vi "QAM Bit Grouping.vi"(1 "BitStream In":i32[](array[numeric]), 2 "QAM Complexity":T1(ring)) -> (0 "Symbol Out":i32[](array[numeric]))   [LabVIEW 2018]
doc: "Converts a binary stream into integer weights for QAM Modulation\nSupports: BPSK, QPSK, 16-QAM, 64-QAM, 256-QAM"
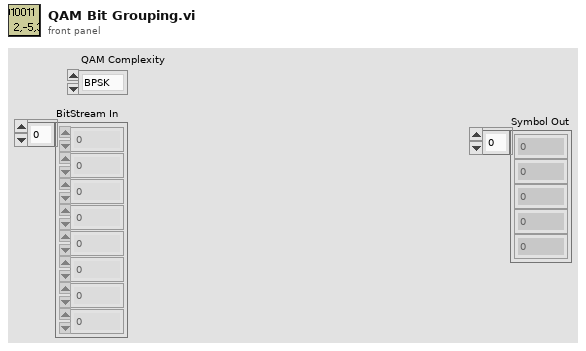
[diagram p1: front panel]
types:
  T1 = enum16{"BPSK", "QPSK", "16-QAM", "64-QAM", "256-QAM"}
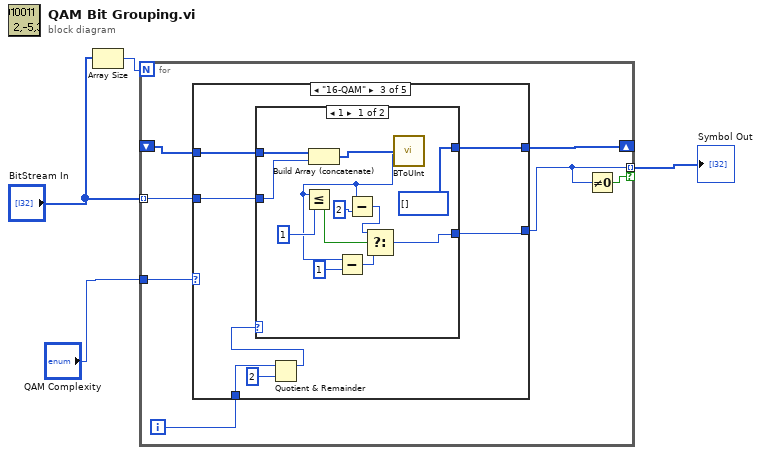
[diagram p0: block diagram]
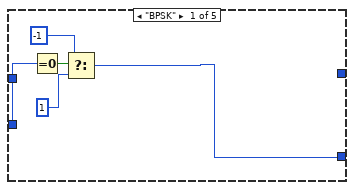
[diagram p2: hidden frame]
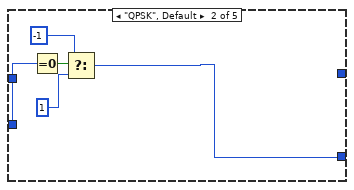
[diagram p3: hidden frame]
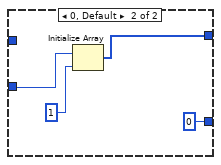
[diagram p4: hidden frame]
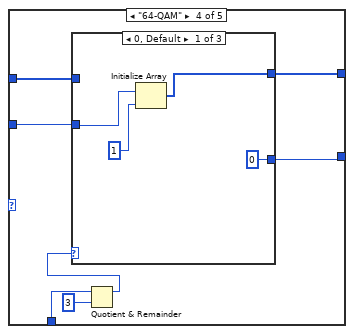
[diagram p5: hidden frame]
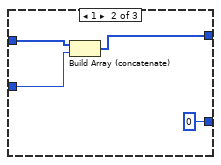
[diagram p6: hidden frame]
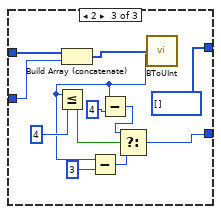
[diagram p7: hidden frame]
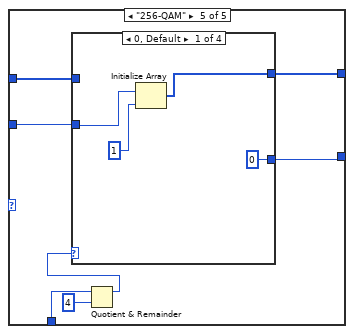
[diagram p8: hidden frame]
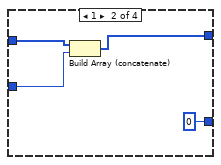
[diagram p9: hidden frame]
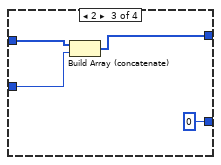
[diagram p10: hidden frame]
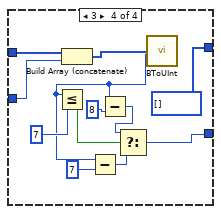
[diagram p11: hidden frame]
diagram:
  n1 = Array Size(array="BitStream In") -> (size(s)=w4:i32)
  n2 = for {
    N: w4 -> [_]
    tunnel: "QAM Complexity" -> [w11]
    tunnel: "BitStream In" -> [w10] mode=indexing
    tunnel: [w7] -> w2 mode=indexing if=w8
    shift-right: [w6] -> _
    shift-left: _ -> [w5]
    i -> [w9]
    n3 = case shown="\"16-QAM\"" w11 {
      tunnel: w10 -> [w16 w21 w26 w49 w76]
      tunnel: w9 -> [_ _ w28 w51 w78]
      tunnel: [w12 w17 w24 w47 w74] -> w7
      tunnel: [_ _ w23 w46 w73] -> w6
      tunnel: w5 -> [_ _ w22 w45 w72]
      frame "BPSK" {
        n4 = Equal To 0?(x=w16) -> (x = 0?=w15:bool)
        n5 = Select(t=-1, s=w15, f=1) -> (s? t:f=w12:i32)
      }
      frame "QPSK", Default {
        n6 = Equal To 0?(x=w21) -> (x = 0?=w20:bool)
        n7 = Select(t=-1, s=w20, f=1) -> (s? t:f=w17:i32)
      }
      frame "16-QAM" {
        n8 = Quotient & Remainder(x=w28, y=2) -> (x-y*floor(x/y)=w25:i32)  [unwired: 1 out]
        n9 = case shown="1" w25 {
          tunnel: w26 -> [w40 w43]
          tunnel: [w31 0] -> w24
          tunnel: [i32[] [] w41] -> w23
          tunnel: w22 -> [w29 _]
          frame 1 {
            n10 = Build Array (concatenate)(w29, w40) -> (w39:i32[])
            n11 = call "BToUInt.vi"("Binary Array"=w39) -> ("Unsigned  Integer"=w34:i32)
            n12 = Less Or Equal?(x=w34, y=1) -> (x <= y?=w37:bool)
            n13 = Subtract(x=w34, y=1) -> (x-y=w32:i32)
            n14 = Subtract(x=w34, y=2) -> (x-y=w35:i32)
            n15 = Select(t=w35, s=w37, f=w32) -> (s? t:f=w31:i32)
          }
          frame 0, Default {
            n16 = Initialize Array(w43, 1 ("dimension size")) -> (w41:i32[])
          }
        }
      }
      frame "64-QAM" {
        n17 = Quotient & Remainder(x=w51, y=3) -> (x-y*floor(x/y)=w48:i32)  [unwired: 1 out]
        n18 = case shown="0, Default" w48 {
          tunnel: w49 -> [w54 w58 w71]
          tunnel: [0 0 w62] -> w47
          tunnel: [w52 w57 i32[] []] -> w46
          tunnel: w45 -> [_ w59 w60]
          frame 0, Default {
            n19 = Initialize Array(w54, 1 ("dimension size")) -> (w52:i32[])
          }
          frame 1 {
            n20 = Build Array (concatenate)(w59, w58) -> (w57:i32[])
          }
          frame 2 {
            n21 = Build Array (concatenate)(w60, w71) -> (w70:i32[])
            n22 = call "BToUInt.vi"("Binary Array"=w70) -> ("Unsigned  Integer"=w65:i32)
            n23 = Less Or Equal?(x=w65, y=4) -> (x <= y?=w68:bool)
            n24 = Subtract(x=w65, y=3) -> (x-y=w63:i32)
            n25 = Subtract(x=w65, y=4) -> (x-y=w66:i32)
            n26 = Select(t=w66, s=w68, f=w63) -> (s? t:f=w62:i32)
          }
        }
      }
      frame "256-QAM" {
        n27 = Quotient & Remainder(x=w78, y=4) -> (x-y*floor(x/y)=w75:i32)  [unwired: 1 out]
        n28 = case shown="0, Default" w75 {
          tunnel: w76 -> [w81 w85 w89 w102]
          tunnel: [0 0 0 w93] -> w74
          tunnel: [w79 w84 w88 i32[] []] -> w73
          tunnel: w72 -> [_ w86 w90 w91]
          frame 0, Default {
            n29 = Initialize Array(w81, 1 ("dimension size")) -> (w79:i32[])
          }
          frame 1 {
            n30 = Build Array (concatenate)(w86, w85) -> (w84:i32[])
          }
          frame 2 {
            n31 = Build Array (concatenate)(w90, w89) -> (w88:i32[])
          }
          frame 3 {
            n32 = Build Array (concatenate)(w91, w102) -> (w101:i32[])
            n33 = call "BToUInt.vi"("Binary Array"=w101) -> ("Unsigned  Integer"=w96:i32)
            n34 = Less Or Equal?(x=w96, y=7) -> (x <= y?=w99:bool)
            n35 = Subtract(x=w96, y=7) -> (x-y=w94:i32)
            n36 = Subtract(x=w96, y=8) -> (x-y=w97:i32)
            n37 = Select(t=w97, s=w99, f=w94) -> (s? t:f=w93:i32)
          }
        }
      }
    }
    n38 = Not Equal To 0?(x=w7) -> (x != 0?=w8:bool)
  }
  "Symbol Out" <- w2
